vi "Event Handle Loop_Draw Integral Button.vi"(8 "error in (no error)":errorcluster, 9 "Button Attribute":T1, 10 "Index":i32, 11 "QMenu Class in":refnum<class "QMenu Class.lvclass">) -> (0 "error out":errorcluster, 2 "Picture":picture, 3 "QMenu Class out":refnum<class "QMenu Class.lvclass">)   [LabVIEW 2020, in "QTab.lvlib" / "QMenu Class.lvclass"]
uses:
  QMenu Class.lvclass
  Button Attribute.ctl
  QMenu Class.lvclass/QMenu Class.ctl
  Read Button Image.vi
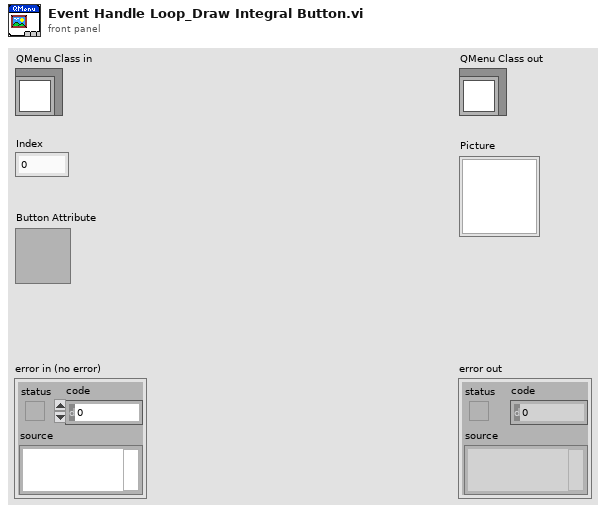
[diagram p1: front panel]
types:
  T1 = typedef "QTab.lvlib/QMenu Class.lvclass/Button Attribute.ctl" = cluster{"Label":string, "Button Text":string, "Closable":bool, "Draggable":bool}
  T2 = typedef "imagedata.ctl" = cluster{"image type":i32, "image depth":i32, "image":u8[], "mask":u8[], "colors":u32[], "Rectangle":cluster{"left":i16, "top":i16, "right":i16, "bottom":i16}}
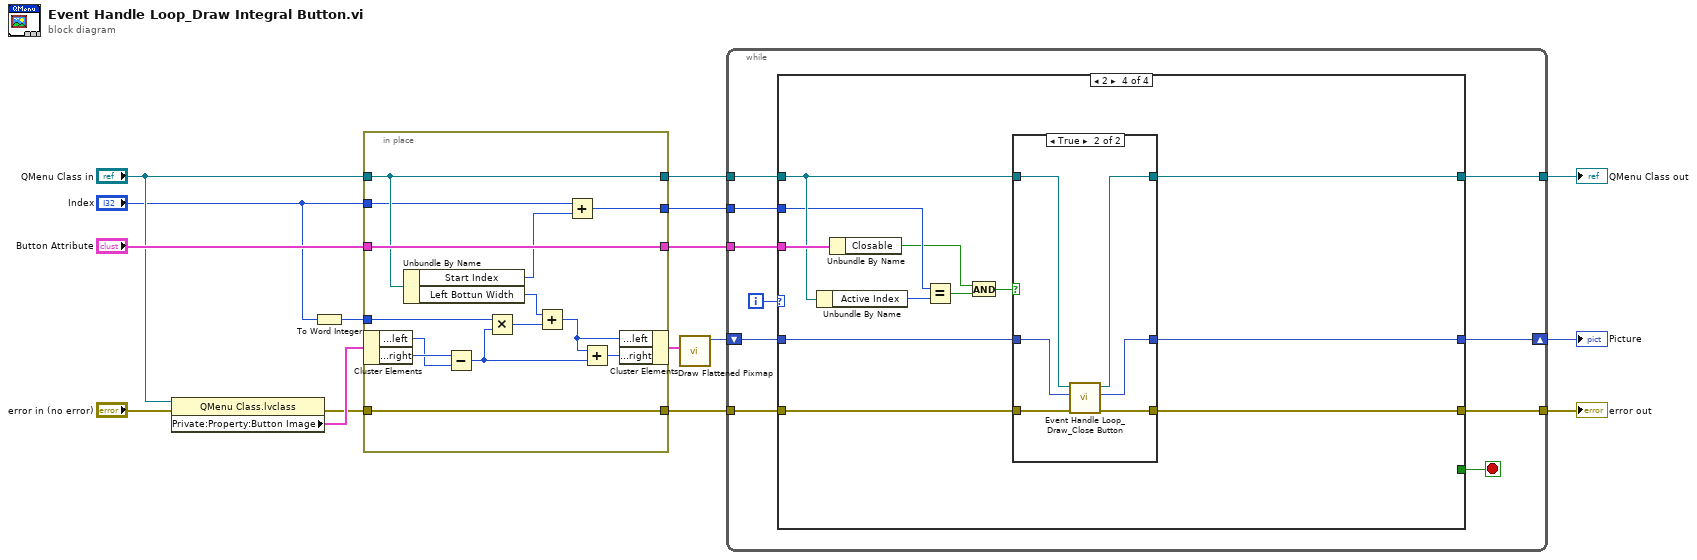
[diagram p0: block diagram]
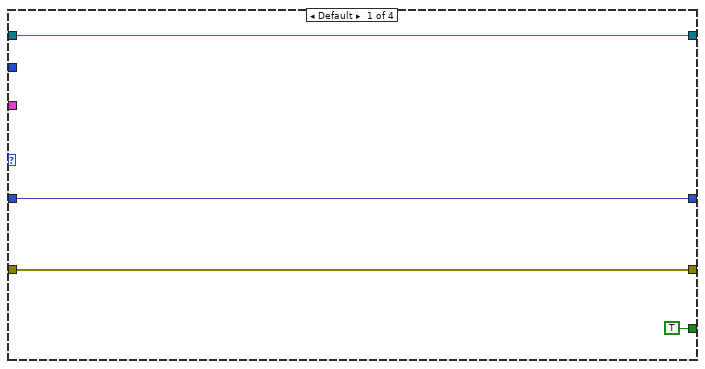
[diagram p2: hidden frame]
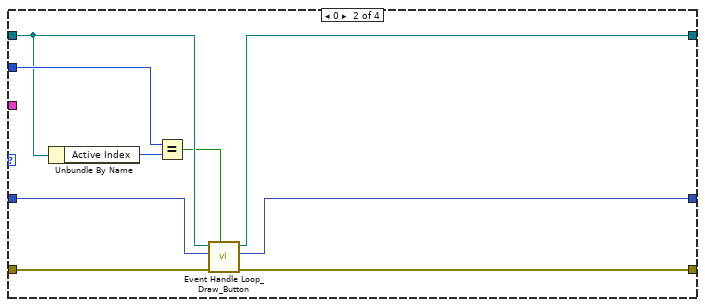
[diagram p3: hidden frame]
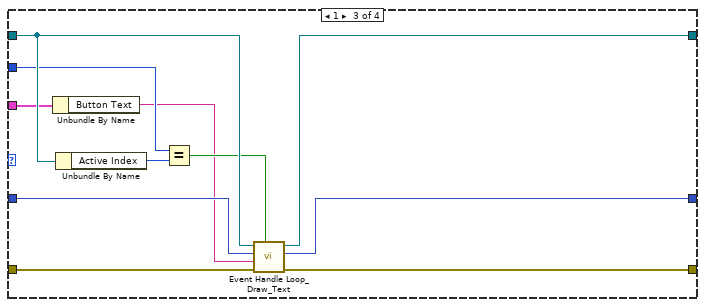
[diagram p4: hidden frame]
diagram:
  n1 = property class="QMenu Class.lvclass"(reference="QMenu Class in", error in="error in (no error)") -> (error out=w11:errorcluster, "Private:Property:Button Image"=w12:T2)  [unwired: 1 out]
  n2 = To Word Integer(number="Index") -> (16bit integer=w7:i16)
  n3 = in-place {
    in-place-border: w7 -> [w28]
    in-place-border: w11 -> [w27]
    in-place-border: [w27] -> w10
    in-place-border: "Button Attribute" -> [w22]
    in-place-border: [w22] -> w5
    in-place-border: [w18] -> w4
    in-place-border: "QMenu Class in" -> [w20]
    in-place-border: [w20] -> w2
    in-place-border: "Index" -> [w17]
    n4 = in-place-cluster #1(w12) -> ("Rectangle.left"=w29:i16, "Rectangle.right"=w30:i16)
    n5 = Unbundle By Name(w20) -> ("Start Index"=w19:i32, "Left Bottun Width"=w21:i16)
    n6 = Subtract(x=w30, y=w29) -> (x-y=w26:i16)
    n7 = Multiply(x=w28, y=w26) -> (x*y=w24:i16)
    n8 = Add(x=w21, y=w24) -> (x+y=w23:i16)
    n9 = Add(x=w17, y=w19) -> (x+y=w18:i32)
    n10 = Add(x=w23, y=w26) -> (x+y=w25:i16)
    n11 = in-place-cluster #1("Rectangle.left"=w23, "Rectangle.right"=w25) -> (w9:T2)
  }
  n12 = call <vilib>:"Draw Flattened Pixmap.vi"("image data"=w9) -> ("new picture"=w8:picture)  [unwired: 8 in]
  n13 = while {
    shift-right: [w36] -> w14
    shift-left: w8 -> [w40]
    tunnel: w5 -> [w38]
    tunnel: w2 -> [w37]
    tunnel: [w35] -> w13
    tunnel: w10 -> [w34]
    tunnel: [w33] -> w15
    tunnel: w4 -> [w31]
    i -> [w39]
    stop <- w32 stop-if-true
    n14 = case shown="2" w39 {
      tunnel: w40 -> [w41 w50 w61 w72]
      tunnel: w38 -> [_ _ w55 w73]
      tunnel: w37 -> [w44 w49 w58 w69]
      tunnel: [w41 w46 w60 w71] -> w36
      tunnel: [w44 w47 w63 w75] -> w35
      tunnel: w34 -> [w43 w51 w64 w76]
      tunnel: [w43 w45 w62 w74] -> w33
      tunnel: [TRUE _ _ _] -> w32
      tunnel: w31 -> [_ w52 w57 w68]
      frame Default {
      }
      frame 0 {
        n15 = Unbundle By Name(w49) -> ("Active Index"=w53:i32)
        n16 = Equal?(x=w52, y=w53) -> (x = y?=w48:bool)
        n17 = call "Event Handle Loop_Draw_Button.vi"("Active"=w48, "error in (no error)"=w51, "Picture In"=w50, "QMenu Class in"=w49) -> ("error out"=w45:errorcluster, "Picture Out"=w46:picture, "QMenu Class out"=w47:refnum<class "QMenu Class.lvclass">)  [unwired: 5 in]
      }
      frame 1 {
        n18 = Unbundle By Name(w55) -> ("Button Text"=w54:string)
        n19 = Unbundle By Name(w58) -> ("Active Index"=w59:i32)
        n20 = Equal?(x=w57, y=w59) -> (x = y?=w56:bool)
        n21 = call "Event Handle Loop_Draw_Text.vi"("Active"=w56, "error in (no error)"=w64, "Text"=w54, "Picture In"=w61, "QMenu Class in"=w58) -> ("error out"=w62:errorcluster, "Picture Out"=w60:picture, "QMenu Class out"=w63:refnum<class "QMenu Class.lvclass">)  [unwired: 4 in]
      }
      frame 2 {
        n22 = Unbundle By Name(w69) -> ("Active Index"=w70:i32)
        n23 = Unbundle By Name(w73) -> ("Closable"=w66:bool)
        n24 = Equal?(x=w68, y=w70) -> (x = y?=w67:bool)
        n25 = And(x=w66, y=w67) -> (x .and. y?=w65:bool)
        n26 = case shown="True" w65 {
          tunnel: w76 -> [w78 w85]
          tunnel: [w77 w84] -> w75
          tunnel: [w78 w83] -> w74
          tunnel: w72 -> [w79 w82]
          tunnel: [w79 w81] -> w71
          tunnel: w69 -> [w77 w80]
          frame False {
          }
          frame True {
            n27 = call "Event Handle Loop_Draw_Close Button.vi"("error in (no error)"=w85, "Picture In"=w82, "QMenu Class in"=w80) -> ("error out"=w83:errorcluster, "Picture Out"=w81:picture, "QMenu Class out"=w84:refnum<class "QMenu Class.lvclass">)  [unwired: 6 in]
          }
        }
      }
    }
  }
  "error out" <- w15
  "QMenu Class out" <- w13
  "Picture" <- w14
